vi "configureAcquisition.vi"(6 "imagePaths":path[](array[path]), 7 "saveImages?":bool, 8 "error in (no error)":errorcluster, 9 "number of Images":i32, 10 "CamaraSettings":refnum<class "CamaraSettings.lvclass">, 11 "NetworkPixelfly in":refnum<class "NetworkPixelfly.lvclass">) -> (0 "error out":errorcluster, 3 "NetworkPixelfly out":refnum<class "NetworkPixelfly.lvclass">)   [LabVIEW 2009, in "Hardware.lvlib" / "HWControllers.lvlib" / "NetworkPixelfly.lvclass"]
uses:
  NetworkPixelfly.lvclass
  Tools/CameraSettings/CamaraSettings.lvclass
  Channels/Camera/PixelflySA/PixelflySA.lvclass
  NetworkPixelfly.lvclass/NetworkPixelfly.ctl
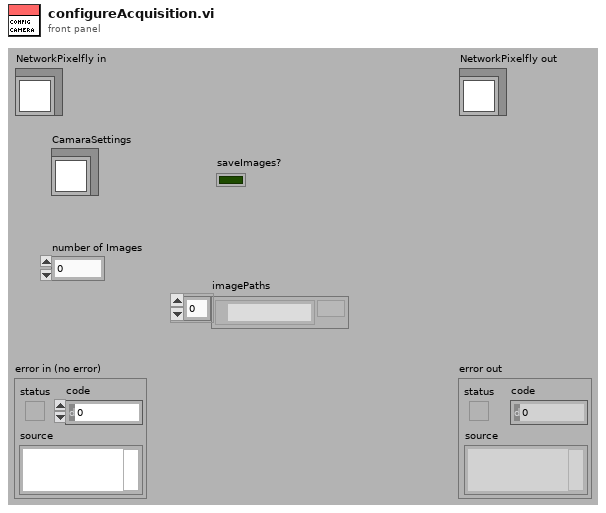
[diagram p1: front panel]
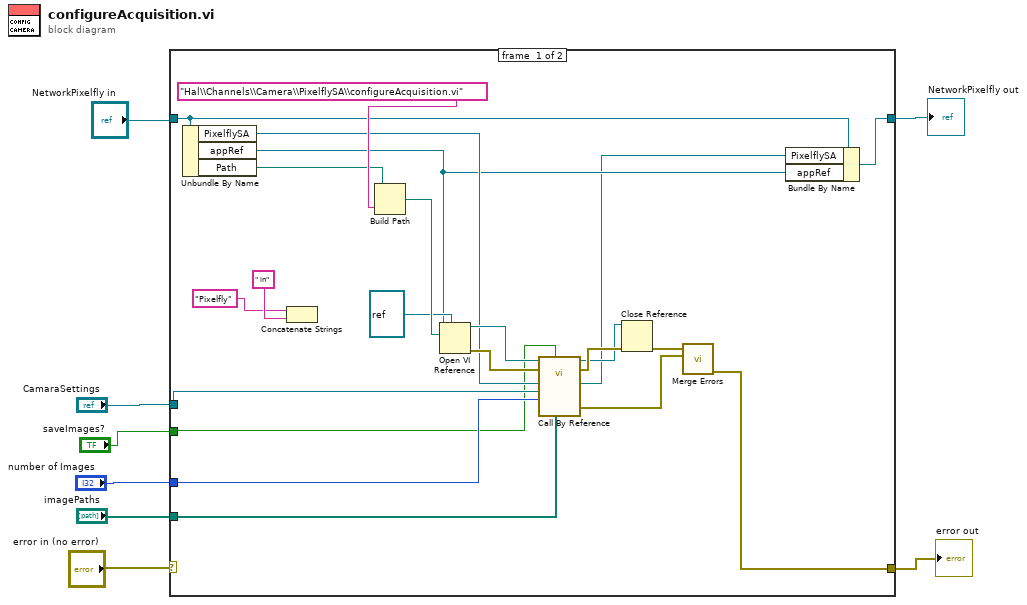
[diagram p0: block diagram]
diagram:
  n1 = case shown="No Error" "error in (no error)" {
    selector: "error in (no error)" -> [_ w32]
    tunnel: [w9 w32] -> w6
    tunnel: [w10 w31] -> w7
    tunnel: "NetworkPixelfly in" -> [w13 w31]
    tunnel: "CamaraSettings" -> [w22 _]
    tunnel: "saveImages?" -> [w19 _]
    tunnel: "number of Images" -> [w20 _]
    tunnel: "imagePaths" -> [w18 _]
    frame #0 {
      n2 = Unbundle By Name(w13) -> ("PixelflySA"=w21:refnum<class "PixelflySA.lvclass">, "appRef"=w12:refnum<vi>, "Path"=w26:path)
      n3 = Concatenate Strings("Pixelfly" ("Control name"), " in") -> ()  [unwired: 1 out]
      n4 = Build Path(base path=w26, name or relative path="Hal\\Channels\\Camera\\PixelflySA\\configureAcquisition.vi" ("viPath")) -> (appended path=w30:path)
      n5 = Open VI Reference(type specifier VI Refnum (for type only)=refnum<vi> refnum, application reference (local)=w12, vi path=w30) -> (vi reference=w23:refnum<vi>, error out=w24:errorcluster)  [unwired: 3 in]
      n6 = call-by-ref "?"(reference=w23, error in=w24, "imagePaths"=w18, "saveImages?"=w19, "number of Images"=w20, "CameraSettings"=w22, "Pixelfly in"=w21) -> (reference out=w16:refnum<vi>, error out=w17:errorcluster, 0:"error out"=w14:errorcluster, "Pixelfly out"=w11:refnum<class "PixelflySA.lvclass">)  [unwired: 5 in]
      n7 = Close Reference(reference=w16, error in (no error)=w17) -> (error out=w15:errorcluster)
      n8 = call <vilib>:"Merge Errors.vi"("error in 2 (no error)"=w14, "error in 1 (no error)"=w15) -> ("error out"=w9:errorcluster)  [unwired: 5 in]
      n9 = Bundle By Name(cluster=w13, "PixelflySA"=w11, "appRef"=w12) -> (w10:refnum<class "NetworkPixelfly.lvclass">)
    }
    frame #1 {
    }
  }
  "error out" <- w6
  "NetworkPixelfly out" <- w7
